vi "Parse All Notes.vi"(8 "error in (no error)":errorcluster, 10 "SR Cluster in":T1 {"Creation Date" format="%<%x>T"; "Last Updated" format="%<%x>T"}, 11 "result string":string) -> (0 "error out":errorcluster, 2 "SR Cluster out":T1 {"Creation Date" format="%<%x>T"; "Last Updated" format="%<%x>T"}, 3 "Array":T3[](array[typedef]) {"Note Date" format="%<%x >T"})   [LabVIEW 2018]
uses:
  Type Defs/SR Note Cluster.ctl
  Type Defs/SR Cluster.ctl
  Type Defs/SR Status.ctl
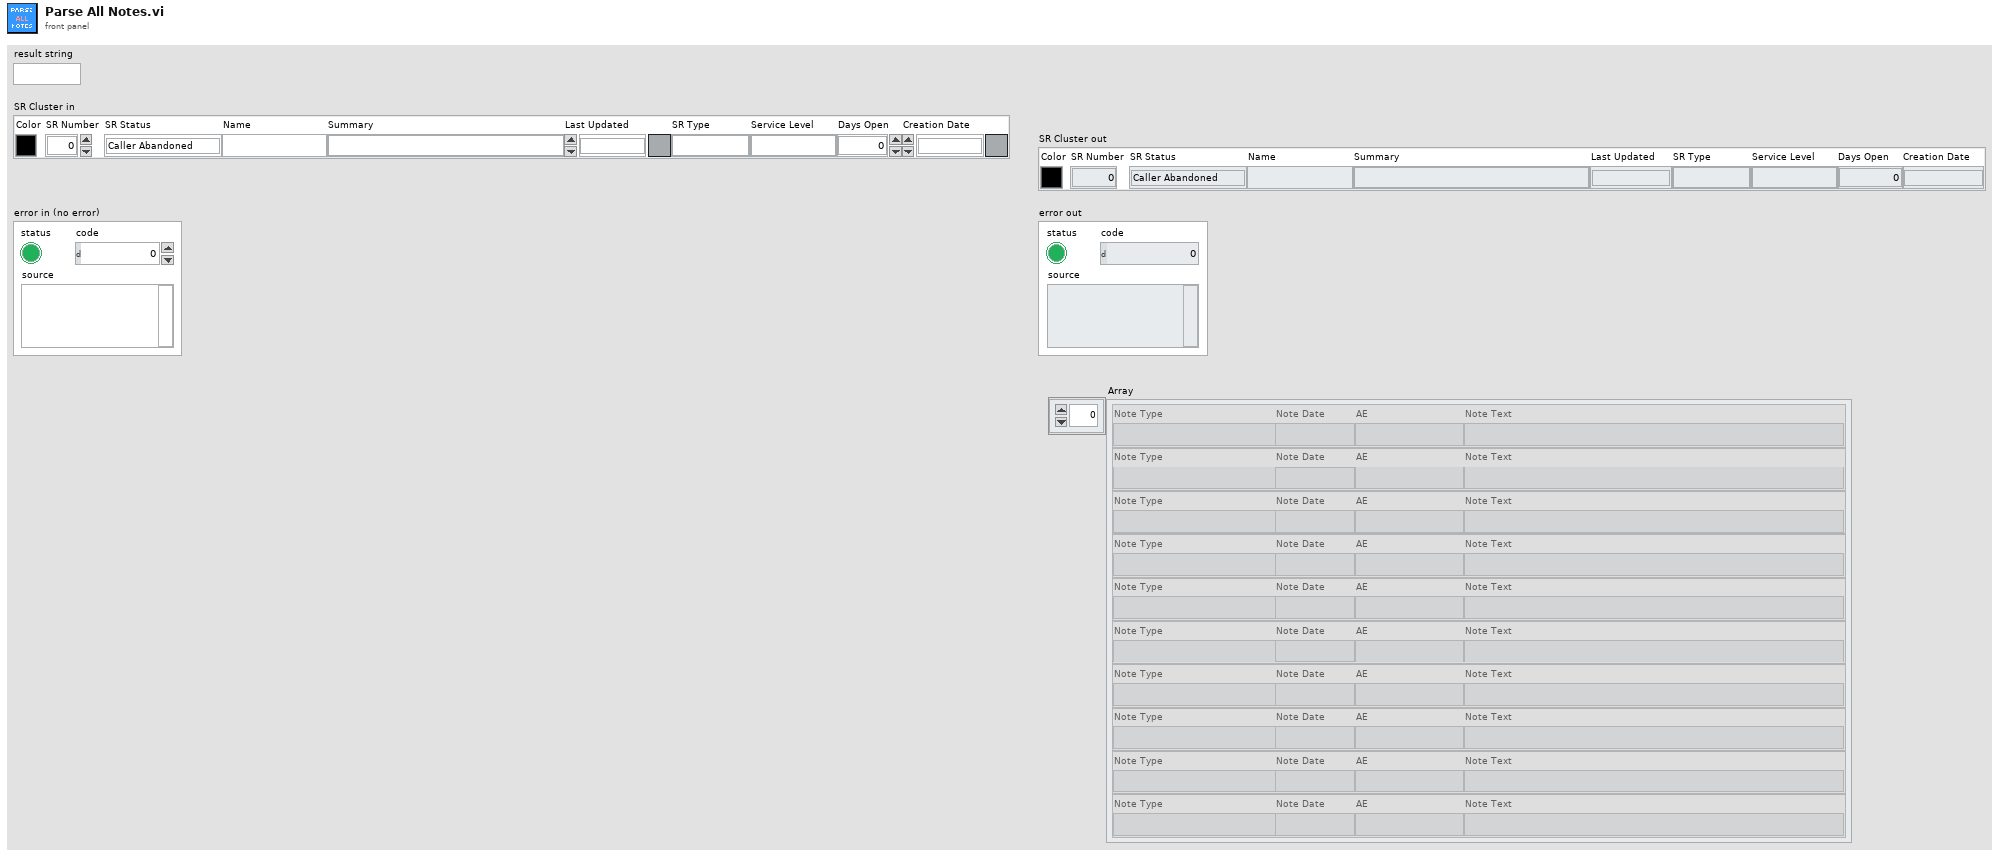
[diagram p1: front panel]
types:
  T1 = typedef "SR Cluster.ctl" = cluster{"Color":u32, "SR Number":i32, "SR Status":T2, "Name":string, "Summary":string, "Last Updated":timestamp, "SR Type":string, "Service Level":string, "Days Open":dbl, "Creation Date":timestamp}
  T2 = typedef "SR Status.ctl" = enum16{"Caller Abandoned", "Created in Error", "Expired", "Forum Resolved AE", "Forum Resolved Customer", "IN WORK", "IN WORK Collab with AES", "IN WORK Collab with PSE", "IN WORK Collab with SE", "IN WORK Customer Added Note", "IN WORK Escalation", "IN WORK Wait on Customer", "Open", "Potentially Resolved", "Presumed Resolved", "RMA Approved for Return", "RMA Closed", "RMA Closed - DOA", "RMA In Progress", "RMA Open", "RMA Waiting on Customer", "Resolved", "Passed Off"}
  T3 = typedef "SR Note Cluster.ctl" = cluster{"Note Type":string, "Note Date":timestamp, "AE":string, "Note Text":string}
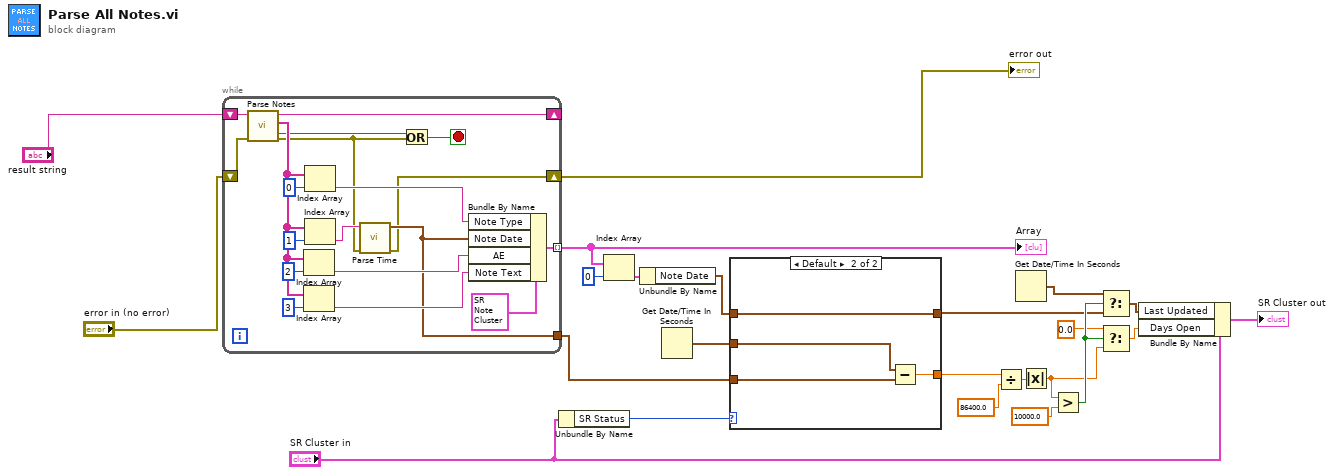
[diagram p0: block diagram]
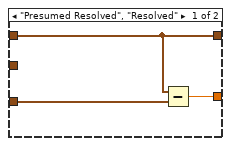
[diagram p2: hidden frame]
diagram:
  n1 = while {
    shift-right: [w41] -> _
    shift-left: "result string" -> [w42]
    tunnel: [w30] -> w17 mode=indexing
    tunnel: [w26] -> w15
    shift-right: [w25] -> w22
    shift-left: "error in (no error)" -> [w40]
    stop <- w29 stop-if-true
    n2 = call "Parse Notes.vi"("error in"=w40, "string in"=w42) -> ("error out"=w24:errorcluster, "Done Reading?"=w28:bool, "sr note out"=w39:string[], "result string out"=w41:string)  [unwired: 6 in]
    n3 = Index Array(array=w39, index=2) -> (element=w32:string)
    n4 = Index Array(array=w39, index=3) -> (element=w33:string)
    n5 = Index Array(array=w39, index=0) -> (element=w31:string)
    n6 = Index Array(array=w39, index=1) -> (element=w27:string)
    n7 = call "Parse Time.vi"("error in (no error)"=w24, "data"=w27) -> ("error out"=w25:errorcluster, "Time Stamp"=w26:timestamp)  [unwired: 8 in]
    n8 = Or(x=w28, y=w24) -> (x .or. y?=w29:bool)
    n9 = Bundle By Name(cluster=T3 {"Note Type"="", "Note Date"=timestamp(0 s since 1904-01-01), "AE"="", "Note Text"=""} ("SR Note Cluster"), "Note Type"=w31, "Note Date"=w26, "AE"=w32, "Note Text"=w33) -> (w30:T3)
  }
  "error out" <- w22
  "Array" <- w17
  n10 = Unbundle By Name("SR Cluster in") -> ("SR Status"=w16:T2)
  n11 = Index Array(array=w17, index=0) -> (element=w19:T3)
  n12 = Unbundle By Name(w19) -> ("Note Date"=w20:timestamp)
  n13 = Get Date/Time In Seconds() -> (seconds since 1Jan1904=w14:timestamp)
  n14 = case shown="Default" w16 {
    tunnel: w20 -> [w45 w46]
    tunnel: w15 -> [w43 w47]
    tunnel: w14 -> [_ w48]
    tunnel: [w44 w49] -> w9
    tunnel: [w45 w46] -> w2
    frame "Presumed Resolved", "Resolved" {
      n15 = Subtract(x=w45, y=w43) -> (x-y=w44:dbl)
    }
    frame Default {
      n16 = Subtract(x=w48, y=w47) -> (x-y=w49:dbl)
    }
  }
  n17 = Divide(x=w9, y=86400.0) -> (x/y=w11:dbl)
  n18 = Get Date/Time In Seconds() -> (seconds since 1Jan1904=w1:timestamp)
  n19 = Absolute Value(x=w11) -> (abs(x)=w3:dbl)
  n20 = Greater?(x=w3, y=10000.0) -> (0:w6:bool)
  n21 = Select(t=w1, s=w6, f=w2) -> (s? t:f=w5:timestamp)
  n22 = Select(t=0.0 ("f"), s=w6, f=w3) -> (s? t:f=w8:dbl)
  n23 = Bundle By Name(cluster="SR Cluster in", "Last Updated"=w5, "Days Open"=w8) -> (→"SR Cluster out":T1)
